vi "ImageAcqControl.vi"(8 "error in (no error)":errorcluster, 10 "Image Acquisition Control Queue":refnum<queue>, 11 "Image in":refnum<class "Image.lvclass">) -> (0 "error out":errorcluster, 2 "Force Stop":bool, 3 "Image out":refnum<class "Image.lvclass">)   [LabVIEW 2012, in "Image.lvclass"]
uses:
  classes/Image.lvclass
  typedefs/ImageViewAcquisitionControl.ctl
  classes/Image.lvclass/Image.ctl
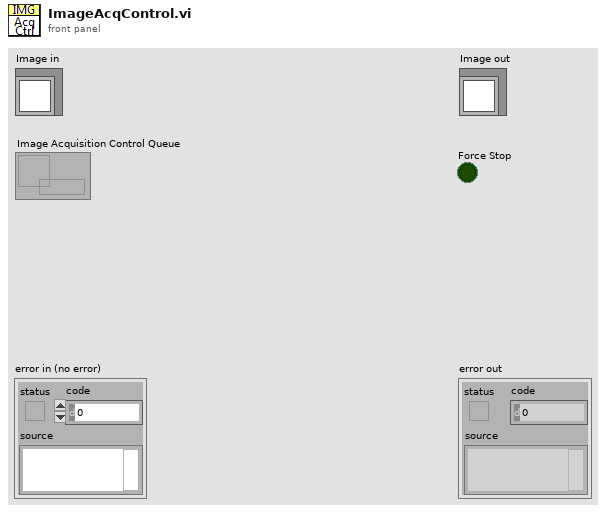
[diagram p1: front panel]
types:
  T1 = typedef "ImageViewAcquisitionControl.ctl" = enum16{"Null", "Stop"}
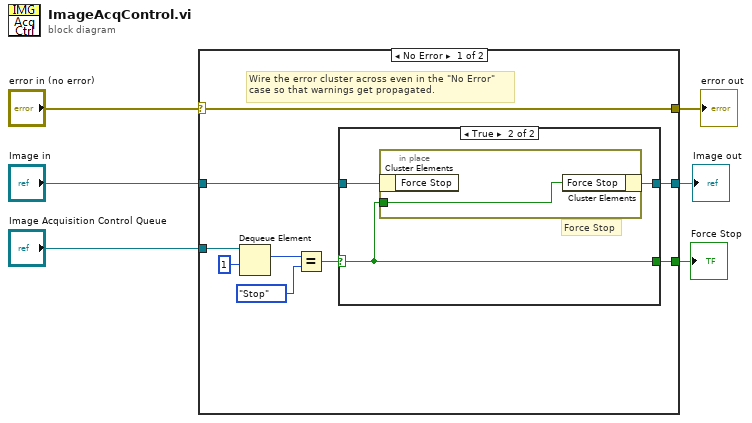
[diagram p0: block diagram]
diagram:
  n1 = case shown="No Error" "error in (no error)" {
    selector: "error in (no error)" -> [w15 w23]
    tunnel: [w15 w23] -> w5
    tunnel: [w9 w22] -> w3
    tunnel: "Image in" -> [w10 w22]
    tunnel: "Image Acquisition Control Queue" -> [w14 _]
    tunnel: [w11 _] -> w1
    frame No Error {
      # "Wire the error cluster across even in the \"No Error\"\ncase so that warnings get propagated."
      n2 = Dequeue Element(queue=w14, timeout in ms (-1)=1) -> (element=w13:T1)  [unwired: 1 in, 3 out]
      n3 = Equal?(x=w13, y=ImageViewAcquisitionControl."Stop") -> (x = y?=w8:bool)
      n4 = case shown="True" w8 {
        selector: w8 -> [w17 w19]
        tunnel: [w17 w19] -> w11
        tunnel: w10 -> [w16 w20]
        tunnel: [w16 w18] -> w9
        frame False {
          # "Continue"
        }
        frame True {
          # "Force Stop"
          n5 = in-place {
            in-place-border: w19 -> [w21]
            n6 = in-place-cluster #1(w20) -> ()  [unwired: 1 out]
            n7 = in-place-cluster #1("Force Stop"=w21) -> (w18:refnum<class "Image.lvclass">)
          }
        }
      }
    }
    frame Error {
    }
  }
  "error out" <- w5
  "Image out" <- w3
  "Force Stop" <- w1
